vi "create T log.vi"(0 "Header String":string="This is a log file of a temperature control run being done in Physics 3600 for the bug experiment. It records the time, temperature, power, and control setting for each PID update. It does so by accumulating the data and periodically saving it.", 2 "create T log":bool, 7 "exp exec in":T1={"data file"={"autosave"=FALSE, "File refnum"=refnum, "data file path"=path ""}, "T log file"={"File refnum"=refnum, "T log file path"=path "", "exists"=FALSE}, "exp seq"={"wave params"={"Num of avg"=0, "Num points"=1000, "Meas rate (Hz)"=100000.0}, "Setpoints"=[], "#"=-1, "index"=-1, "elapsed time (s)"=0.0, "set time (s)"=0.0, "min settle (s)"=30.0, " Exec Status"=enum."Settling"}, "error"={"status"=FALSE, "code"=0, "source"=""}}) -> (4 "exists":bool=TRUE, 8 "exp exec out":T1={"data file"={"autosave"=FALSE, "File refnum"=refnum, "data file path"=path ""}, "T log file"={"File refnum"=refnum, "T log file path"=path "", "exists"=FALSE}, "exp seq"={"wave params"={"Num of avg"=0, "Num points"=1000, "Meas rate (Hz)"=100000.0}, "Setpoints"=[], "#"=-1, "index"=-1, "elapsed time (s)"=0.0, "set time (s)"=0.0, "min settle (s)"=30.0, " Exec Status"=enum."Settling"}, "error"={"status"=FALSE, "code"=0, "source"=""}})   [LabVIEW 2019]
doc: "This is a Bug C(T) subVI.\n\nThis vi prompts the user to choose whether to create a temp data log. If the user so chooses, a temp parameters log file is created with the given header.\n\nPaul K Dixon\nPhysics 3600\nCSUSB Physics"
uses:
  typedefs/PID exec cluster.ctl
  typedefs/data file info.ctl
  typedefs/bug temp file info.ctl
  typedefs/exp seq cluster.ctl
  typedefs/wvfm acq params.ctl
  typedefs/bug meas status.ctl
  globals/Bug globals.vi
panel:
  out "temp log file path":path
  in  "String":string="Time (ms)\tTemp (C)\tPower\tSetpoint\tCB\tItime\tIon\tDtime\tDon\tSB\tStime\tTime in SB\tSettled\tMan Pow\tMan on"
  out "file refnum out":refnum<file>
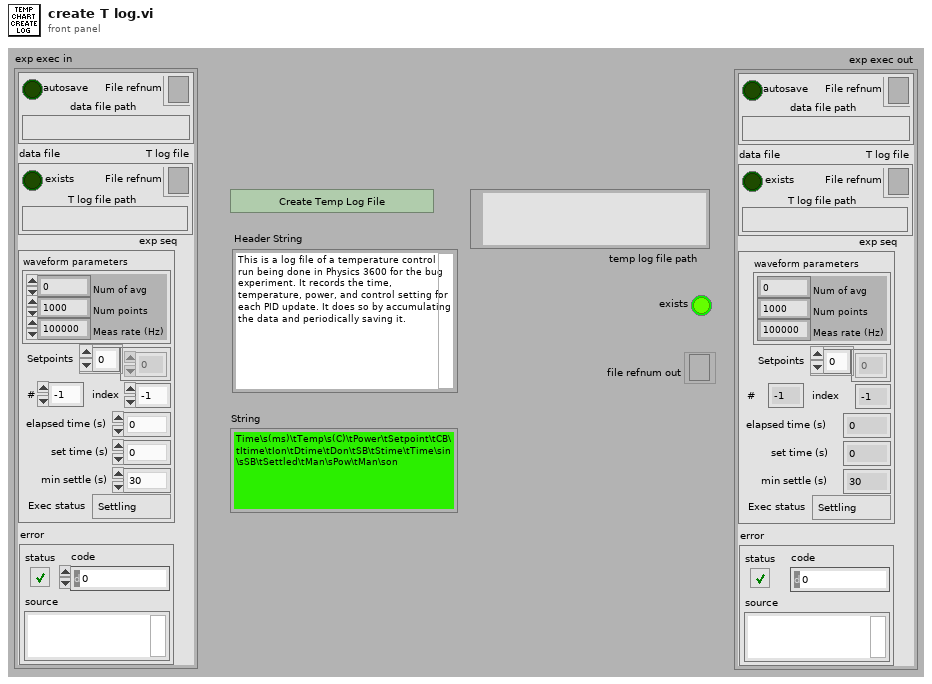
[diagram p1: front panel]
types:
  T1 = typedef "PID exec cluster.ctl" = cluster{"data file":T2, "T log file":T3, "exp seq":T4, "error":errorcluster}
  T2 = typedef "data file info.ctl" = cluster{"autosave":bool, "File refnum":refnum<file>, "data file path":path}
  T3 = typedef "bug temp file info.ctl" = cluster{"File refnum":refnum<file>, "T log file path":path, "exists":bool}
  T4 = typedef "exp seq cluster.ctl" = cluster{"wave params":T5, "Setpoints":dbl[], "#":i32, "index":i32, "elapsed time (s)":dbl, "set time (s)":dbl, "min settle (s)":dbl, " Exec Status":T6}
  T5 = typedef "wvfm acq params.ctl" = cluster{"Num of avg":i32, "Num points":i32, "Meas rate (Hz)":dbl}
  T6 = typedef "bug meas status.ctl" = enum32{"Settling", "Measuring", "Holding", "Exit"}
  T7 = typedef "temp cont cluster.ctl" = cluster{"T exec":T8, "T status":T10, "T params":T12, "utility":T13}
  T8 = typedef "temp exec cluster.ctl" = cluster{"T mode":T9, "exec setpoint":dbl, "reset":bool, "man power":dbl, "man":bool, "log":bool, "clear":bool}
  T9 = typedef "temp mode enum.ctl" = enum16{"settling", "measuring", "holding", "Exit"}
  T10 = typedef "temp indicator.ctl" = cluster{"Control status":T11, "Temp":dbl, "Power":dbl, "Time in settle band":dbl, "Settled":bool, "Low":bool, "High":bool, "Setpoint":dbl, "Control":bool, "In Settle Band":bool}
  T11 = typedef "temp control status.ctl" = enum16{"In Settle Band", "In Control Band", "Below Control Band", "Above Control Band"}
  T12 = typedef "PID control parameters.ctl" = cluster{"Setpoint":dbl, "Control Bandwidth":dbl, "Integral Time":dbl, "Int\nON":bool, "Derivative Tme":dbl, "Der\nON":bool, "Settle Bandwidth":dbl, "Settle Time":dbl}
  T13 = typedef "temp cont utility.ctl" = cluster{"meas index":i32, "wait (ms)":i32, "H Vmax":dbl, "power out":dbl, "heat volt out":dbl, "heat volt in":dbl, "therm volt":dbl, "t T P hist":dbl[][], "cont hist":dbl[][]}
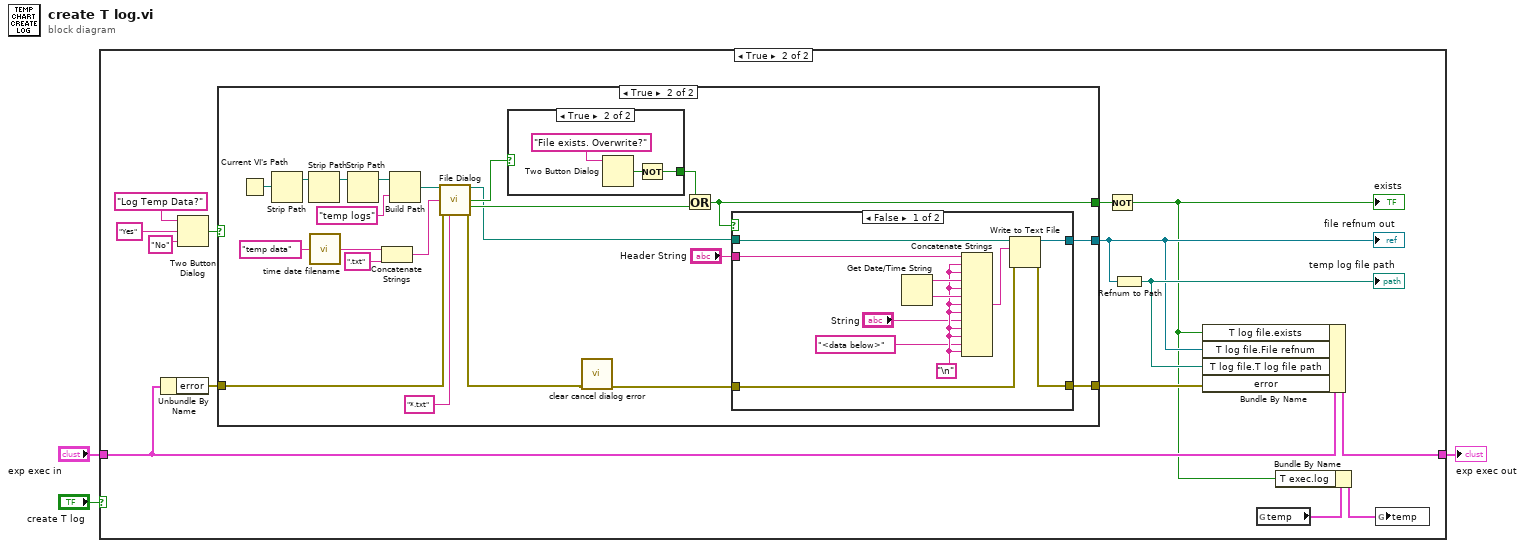
[diagram p0: block diagram]
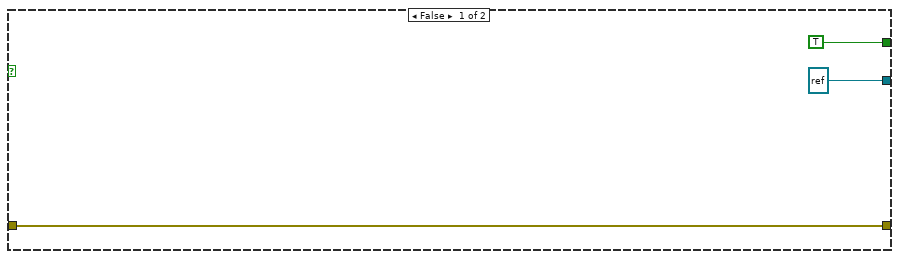
[diagram p3: hidden frame]
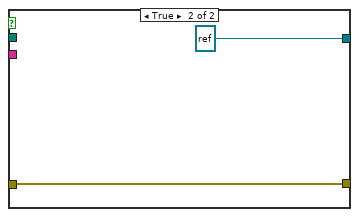
[diagram p4: hidden frame]
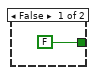
[diagram p5: hidden frame]
diagram:
  n1 = case shown="True" "create T log" {
    tunnel: "exp exec in" -> [w4 w13]
    tunnel: [w4 w11] -> w2
    frame False {
    }
    frame True {
      n2 = Unbundle By Name(w13) -> ("error"=w12:errorcluster)
      n3 = Two Button Dialog(message="Log Temp Data?", 1:"No" ("F button name (\"Cancel\")"), 2:"Yes" ("T button name (\"OK\")")) -> (T button?=w14:bool)
      n4 = case shown="True" w14 {
        tunnel: [TRUE w39] -> w18
        tunnel: [w21 w37] -> w10
        tunnel: [refnum<file> refnum ("refnum out") w36] -> w8
        tunnel: w12 -> [w21 w34]
        frame False {
        }
        frame True {
          n5 = Current VI's Path() -> (path=w42:path)
          n6 = Strip Path(path=w42) -> (stripped path=w43:path)  [unwired: 1 out]
          n7 = Strip Path(path=w43) -> (stripped path=w29:path)  [unwired: 1 out]
          n8 = call "time date filename.vi"("file name in"="temp data" ("name or relative path")) -> ("time date file name out"=w24:string)  [unwired: 14 in]
          n9 = Strip Path(path=w29) -> (stripped path=w28:path)  [unwired: 1 out]
          n10 = Concatenate Strings(w24, ".txt" ("name or relative path")) -> (w22:string)
          n11 = Build Path(base path=w28, name or relative path="temp logs") -> (appended path=w26:path)
          n12 = call "File Dialog"("start path"=w26, "default name"=w22, "error in"=w34, "pattern (all files)"="*.txt") -> ("selected path"=w31:path, "exists"=w33:bool, "cancelled"=w32:bool, "error out"=w30:errorcluster)  [unwired: 8 in]
          n13 = case shown="True" w33 {
            tunnel: [FALSE ("T button?") w58] -> w41
            frame False {
            }
            frame True {
              n14 = Two Button Dialog(message="File exists. Overwrite?") -> (T button?=w59:bool)  [unwired: 2 out]
              n15 = Not(x=w59) -> (.not. x?=w58:bool)
            }
          }
          n16 = call "clear cancel dialog error.vi"("error in"=w30) -> ("error out"=w38:errorcluster)  [unwired: 14 out]
          n17 = Or(x=w41, y=w32) -> (x .or. y?=w39:bool)
          n18 = case shown="False" w39 {
            tunnel: "Header String" -> [w47 _]
            tunnel: w31 -> [w53 _]
            tunnel: w38 -> [w52 w55]
            tunnel: [w51 w55] -> w37
            tunnel: [w50 refnum<file> refnum ("refnum out")] -> w36
            frame False {
              w46 = "\n"
              n19 = Get Date/Time String() -> (date string=w49:string, time string=w48:string)  [unwired: 3 in]
              n20 = Concatenate Strings(w47, w46, w46, w49, w46, w48, w46, w46, "String", w46, w46, "<data below>", w46) -> (w54:string)
              n21 = Write to Text File(file (use dialog)=w53, text=w54, error in=w52) -> (refnum out=w50:refnum<file>, error out=w51:errorcluster)  [unwired: 2 out]
            }
            frame True {
            }
          }
        }
      }
      "file refnum out" <- w8
      n22 = Not(x=w18) -> (.not. x?=w5:bool)
      "exists" <- w5
      n23 = Refnum to Path(1:w8) -> (0:w9:path)
      "temp log file path" <- w9
      n24 = Bundle By Name(cluster=w13, "T log file.exists"=w5, "T log file.File refnum"=w8, "T log file.T log file path"=w9, "error"=w10) -> (w11:T1)
      n25 = global read "Bug globals.vi" "temp"() -> (w7:T7)
      n26 = Bundle By Name(cluster=w7, "T exec.log"=w5) -> (w6:T7)
      n27 = global write "Bug globals.vi" "temp"(w6) -> ()
    }
  }
  "exp exec out" <- w2
